vi "2D Cartesian Coordinate Shift (Scalar).vi"(8 "shift":cluster{"dx":dbl, "dy":dbl}, 10 "y":dbl, 11 "x":dbl) -> (0 "error":i32, 2 "y out":dbl, 3 "x out":dbl)   [LabVIEW 2020, in "NI_AALPro.lvlib"]
doc: "Shifts two-dimensional Cartesian coordinates along the x- and y-axes. Wire data to the <B>X</B> input to determine the polymorphic instance to use or manually select the instance."
uses:
  <vilib>/Analysis/NI_AALPro.lvlib
  <resource>/lvanlys.dll
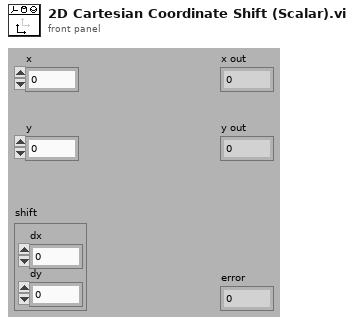
[diagram p1: front panel]
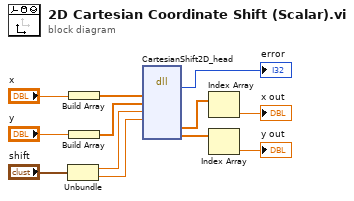
[diagram p0: block diagram]
diagram:
  n1 = Unbundle("shift") -> ("dx"=w7:dbl, "dy"=w6:dbl)
  n2 = Build Array("x") -> (w11:dbl[])
  n3 = Build Array("y") -> (w9:dbl[])
  n4 = dll-call lib="e:/builds/penguin/labview/branches/2020/dev/dist/resource/lvanlys.*" fn="CartesianShift2D_head"("X"=w11, "Y"=w9, "dx"=w7, "dy"=w6) -> (→"error":i32, "Xout"=w5:dbl[], "Yout"=w3:dbl[])  [unwired: 9 in, 2 out]
  n5 = Index Array(array=w5) -> (element=→"x out":dbl)  [unwired: 1 in]
  n6 = Index Array(array=w3) -> (element=→"y out":dbl)  [unwired: 1 in]
